vi "Dashboard Main.vi"() -> ()   [LabVIEW 2023]
uses:
  <vilib>/event_ctls.llb/eventvkey.ctl
  <vilib>/Rock Robotics/WPI/Dashboard/WPI_DashboardLogging Global.vi
  <vilib>/Rock Robotics/Network Tables/NT Read Numeric Array.vi
  <vilib>/Rock Robotics/Network Tables/NT Read Boolean.vi
panel:
  in  "Camera Settings Right":T1={"Frame Rate"=30, "Compression"=30, "Size"=1, "DB Camera Config"=FALSE} {"Frame Rate" scale=1.0..30.0; "Compression" scale=100.0..-1.0; "Size" items=["640x480", "320x240", "160x120"]}
  in  "Camera Name Right":string(combo)="No Camera Selection"
  out "Camera Perf":string
  in  "Camera Settings":T1={"Frame Rate"=30, "Compression"=30, "Size"=1, "DB Camera Config"=FALSE} {"Frame Rate" scale=1.0..30.0; "Compression" scale=100.0..-1.0; "Size" items=["640x480", "320x240", "160x120"]}
  in  "TCP":refnum<k5>
  in  "Rec Mode":enum32{"Stop", "Record", "Playback"}(radio)
  out "Robot IP":string
  out "Image Message":string="Timeout in Camera Communications"
  in  "Dashboard Tab":T2(tab)=enum."Custom"
  in  "Select Auto":string(combo)="Select Autonomous ..."
  out "NT Connection":bool
  out "MotorChart R":cluster{"Numeric":dbl, "Numeric":dbl}(graph)
  out "MotorChart L":cluster{"Numeric":dbl, "Numeric":dbl}(graph)
  out "MotorSliders R":cluster{"MotorSlide1":dbl, "MotorSlide2":dbl} {"MotorSlide2" scale=-1.0..1.0 scale format="%#_2e"; "MotorSlide1" scale=-1.0..1.0 scale format="%#_2e"}
  out "MotorSliders L":cluster{"MotorSlide1":dbl, "MotorSlide2":dbl} {"MotorSlide2" scale=-1.0..1.0 scale format="%#_2e"; "MotorSlide1" scale=-1.0..1.0 scale format="%#_2e"}
  out "Gyro":dbl(knob) scale=0.0..360.0
  out "JS1 Z":dbl(slide) scale=-1.0..1.0 scale format="%#_2e"
  out "JS1 Graph":cluster{"X":dbl, "Y":dbl}[](graph)
  out "JS1 Buttons":T3
  out "JS2 Z":dbl(slide) scale=-1.0..1.0 scale format="%#_2e"
  out "JS2 Graph":cluster{"X":dbl, "Y":dbl}[](graph)
  out "JS2 Buttons":T3
  out "Mode":T4(ring)=enum."Auto Disabled"
  out "Right Camera Perf":cluster{"Bandwidth (Mbps)":dbl, "FPS":dbl}
  out "Camera Image Right":T5(plugin-control)
  in  "DB/String 9":string
  in  "DB/String 8":string
  in  "DB/String 7":string
  in  "DB/String 6":string
  in  "DB/String 5":string
  in  "DB/String 4":string
  in  "DB/String 3":string
  in  "DB/String 2":string
  in  "DB/String 1":string
  in  "DB/String 0":string
  in  "DB/Slider 0":dbl(slide) scale=0.0..5.0
  in  "DB/Slider 1":dbl(slide) scale=0.0..5.0
  in  "DB/Slider 2":dbl(slide) scale=0.0..5.0
  in  "DB/Slider 3":dbl(slide) scale=0.0..5.0
  out "DB/LED 3":bool
  out "DB/LED 2":bool
  out "DB/LED 1":bool
  out "DB/LED 0":bool
  in  "DB/Button 3":bool
  in  "DB/Button 2":bool
  in  "DB/Button 1":bool
  in  "DB/Button 0":bool caption="New Name"
  out "Cluster":T6
  in  "Test Slider":dbl(slide) scale=0.0..100.0 scale format="%#_3g"
  in  "On/Off":bool caption="Solenoid"
  in  "Test Name":u16(ring) items=["Select the test to run..."]
  in  "Test Tree":string(tree)
  in  "Motor":cluster{"Value":dbl, "Enable":bool} {"Value" scale=-1.0..1.0 scale format="%#_3g"}
  out "Progress":T7 {"Test Progress" scale=0.0..100.0}
  in  "Rev/Fwd":cluster{"Forward":bool, "Reverse":bool}
  in  "Test Ring":u16(ring) items=["Monochrome", "Color"]
  in  "CheckList":i32(listbox)
  out "Tree":string(tree)
  out "Camera Image":T5(plugin-control)
  out "Background":bool
  in  "Camera Name":string(combo)="No Camera Selection"
  # "HW"
  # "HW"
  # "Joysticks"
  # "Drive Motors"
  # "Front"
  # "Right"
  # "Left"
  # "Back"
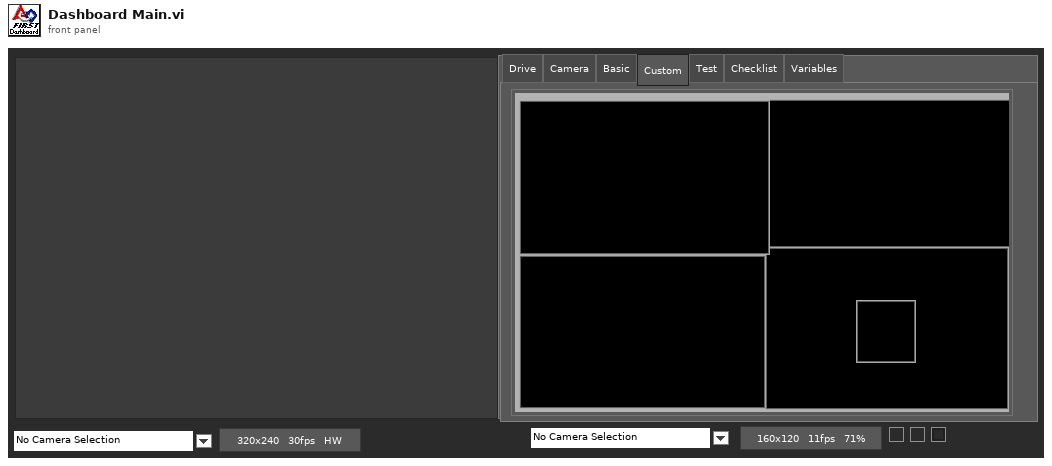
[diagram p1: front panel]
types:
  T1 = cluster{"Frame Rate":i32, "Compression":i32, "Size":u16, "DB Camera Config":bool}
  T2 = enum32{"Drive", "Camera", "Basic", "Custom", "Test", "Checklist", "Variables"}
  T3 = cluster{bool, bool, bool, bool, bool, bool, bool, bool, bool, bool, bool, bool}
  T4 = enum8{"Tele-Op Disabled", "Tele-Op Enabled", "Auto Disabled", "Auto Enabled", "Test Disabled", "Test Enabled", "Disconnected", "No Code", "E-Stop"}
  T5 = typedef "IMAQ Image.ctl" = refnum<image>
  T6 = cluster{"Rotation Align":u32, "Rotation Align 2":u32, "Note Ready":u32, "Y pressed":u32, "Teeth Note":u32}
  T7 = cluster{"Test Progress":u8, "Test Progress Text":string}
  T8 = cluster{"Save Path":path, "Interval (s)":dbl, "Keep":i32}
  T9 = enum32{"Drive", "Camera", "Basic", "Custom", "Test", "Commands", "Checklist", "Variables"}
  T10 = typedef "Image Type" = u32
  T11 = cluster{"Error Strings":string, "Disable Counts":cluster{u16, u16}, "Rail Faults":cluster{u16, u16, u16}, "Robot IP":string, "DB Mode":u8, "Event Info":cluster{"Name":string, "Type":u8, "Number":u16, "Replay":u8}}
  T12 = cluster{"Storage":cluster{"Disk Free":u64, "RAM Block":u32, "RAM free":u32}, "CPU Utilization":cluster{"CPU % ISR":sgl, "CPU % Time Crit":sgl, "CPU % Timed Str":sgl, "CPU % High":sgl, "CPU % Above":sgl, "CPU % Normal":sgl, "CPU % Low":sgl}, "CAN":cluster{"% Bus Utilization":sgl, "Bus Off Cnt":u32, "TX_FIFO Full Cnt":u32, "Receive Error Cnt":u8, "Transmit Error Cnt":u8}, "HID":cluster{"HID Outputs":u32, "Rumble Low":u16, "Rumble High":u16}[]}
  T13 = cluster{"Status bits":cluster{"Test Mode":bool, "Autonomous":bool, "Enabled":bool, "Code Start":bool, "Brownout":bool, "Reserved 2":bool, "Reserved 3":bool, "E-Stop":bool}, "Code Trace":cluster{"Disabled":bool, "TeleOp":bool, "Auto":bool, "Test":bool}, "Controller Type":enum16{"unknown", "cRIO", "roboRio"}, "Code?":enum16{"unknown", "noCode", "code"}, "Battery V":dbl}
  T14 = cluster{"Control Bits":cluster{"TestMode":bool, "Autonomous":bool, "Enabled":bool, "FMS Present":bool, bool, bool, bool, "E-Stop":bool}, "Team Station ":u8, "Countdown":sgl, "Joystick Values":cluster{"Axes":dbl[], "Buttons":bool[], "POVs":i16[]}[]}
  T15 = cluster{"Axes":dbl[], "Buttons":bool[], "POVs":i16[]}[]
  T16 = cluster{"Aligned":u32, "Aligned":u32, "Aligned":u32, "Aligned":u32, "Aligned":u32}
  T17 = cluster{"Axes":dbl[], "Buttons":bool[], "POVs":i16[]}
  T18 = cluster{"Buttons[0]":bool, "Buttons[1]":bool, "Buttons[2]":bool, "Buttons[3]":bool, "Buttons[4]":bool, "Buttons[5]":bool, "Buttons[6]":bool, "Buttons[7]":bool, "Buttons[8]":bool, "Buttons[9]":bool, "Buttons[10]":bool, "Buttons[11]":bool}
  T19 = cluster{"Camera Image":refnum<vi>, "Dashboard Tab":refnum<vi>, "Background":refnum<vi>, "Rec Mode":refnum<vi>, "Test Slider":refnum<vi>, "On/Off ":refnum<vi>, "Test Ring":refnum<vi>, "Rev/Fwd":refnum<vi>, "Test Name":refnum<vi>, "Motor":refnum<vi>, "Progress":refnum<vi>, "CheckList":refnum<vi>, "Tree":refnum<vi>, "Test Tree":refnum<vi>, "Camera Settings":refnum<vi>, "Camera Name":refnum<vi>, "Camera Perf":refnum<vi>, "Camera Settings Right":refnum<vi>, "Camera Name Right":refnum<vi>, "Camera Image Right":refnum<vi>, "Cluster":refnum<vi>}
  T20 = cluster{"Global Rectangle":i32[], "Contours":cluster{"Contour Type":u32, "ROI Type":u32, "Points":i32[]}[]}
  T21 = cluster{"Camera Name":string, string, "Saved DB Images Info":cluster{"Save Path":path, "Interval (s)":dbl, "Keep":i32}}
  T22 = cluster{"Camera Name Right":string, string, "Saved DB Images Info":cluster{"Save Path":path, "Interval (s)":dbl, "Keep":i32}}
  T23 = cluster{"Operation":enum16{"Update", "Clear"}, "Color Box":u32}[]
  T24 = typedef "eventvkey.ctl" = enum16{"ASCII", "Enter", "Return", "Shift", "Ctrl", "Alt", "Cmd", "Opt", "Caps", "NumLock", "Clear", "Break", "Up", "Down", "Left", "Right", "Insert", "Delete", "Home", "End", "PageUp", "PageDown", "Escape", "Help", "Pause", "ScrollLock", "F1", "F2", "F3", "F4", "F5", "F6", "F7", "F8", "F9", "F10", "F11", "F12", "F13", "F14", "F15", "F16", "F17", "F18", "F19", "F20", "F21", "F22", "F23", "F24", "Play", "VolumeUp", "VolumeDown", "Mute", "Two Byte Char"}
  T25 = cluster{"Image Size":bool, "Image Type":bool, "Pixel Value":bool, "ROI Information":bool, "Zoom Factor":bool}
  T26 = cluster{"Operation":enum16{"Update", "Clear"}, "Color Box":u32}
  T27 = cluster{"Shift":bool, "Ctrl":bool, "Alt":bool, "Cmd":bool, "Opt":bool}
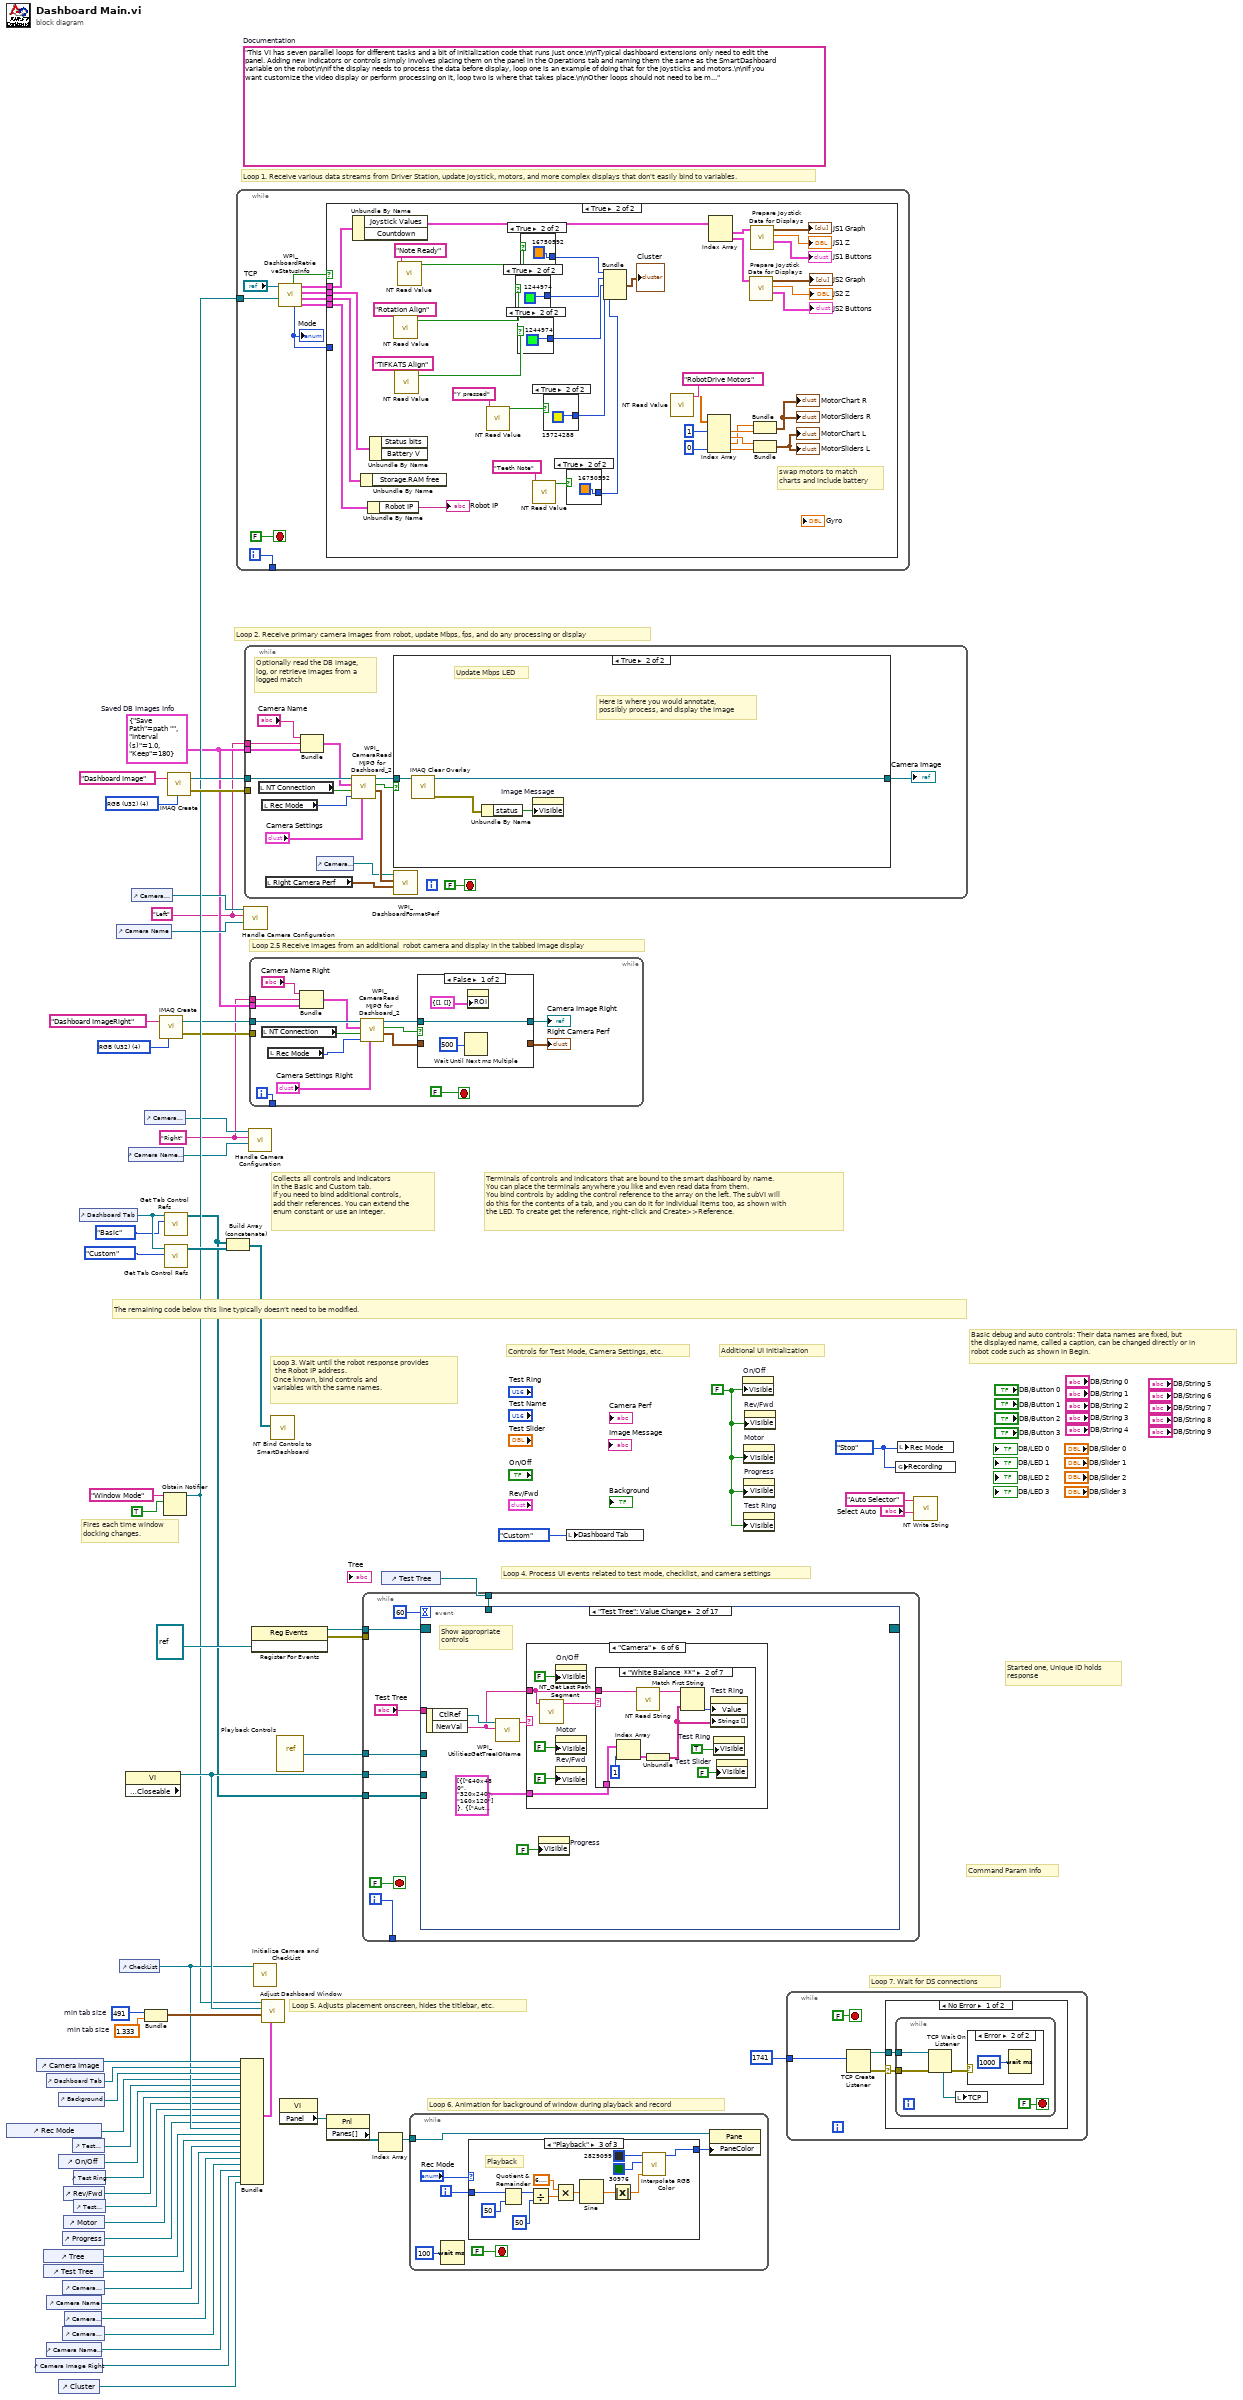
[diagram p0: block diagram]
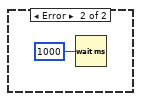
[diagram p4: hidden frame]
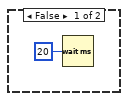
[diagram p5: hidden frame]
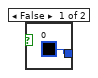
[diagram p6: hidden frame]
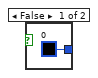
[diagram p7: hidden frame]
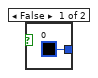
[diagram p8: hidden frame]
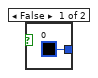
[diagram p9: hidden frame]
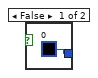
[diagram p10: hidden frame]
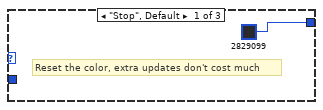
[diagram p11: hidden frame]
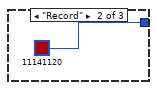
[diagram p12: hidden frame]
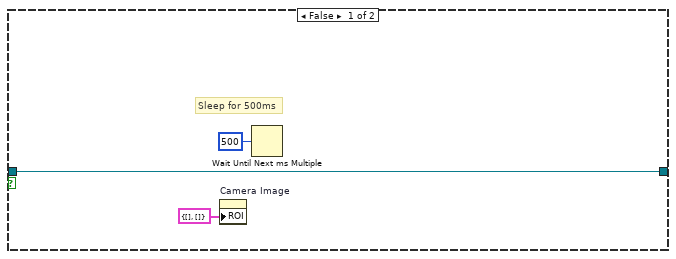
[diagram p13: hidden frame]
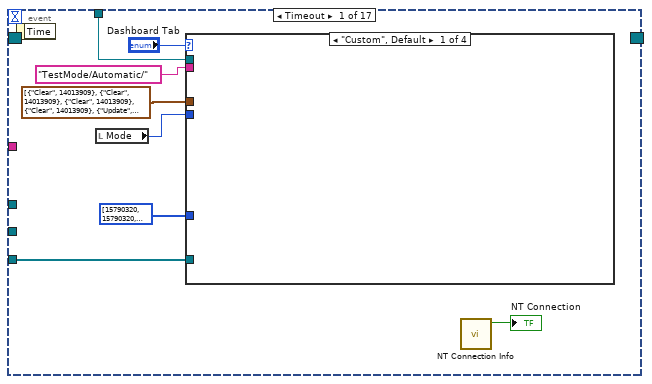
[diagram p14: hidden frame]
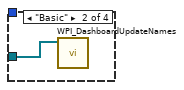
[diagram p15: hidden frame]
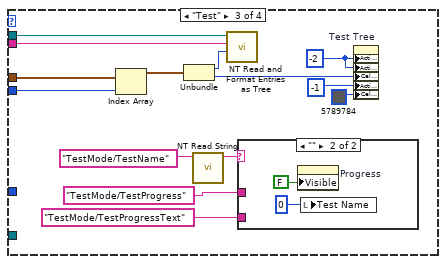
[diagram p16: hidden frame]
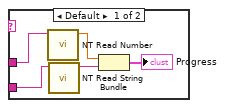
[diagram p17: hidden frame]
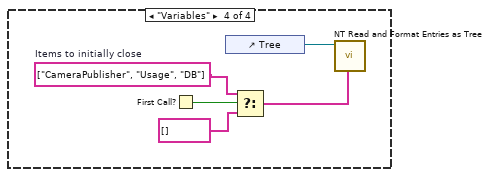
[diagram p18: hidden frame]
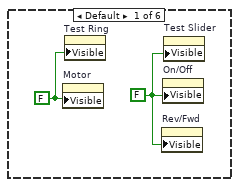
[diagram p19: hidden frame]
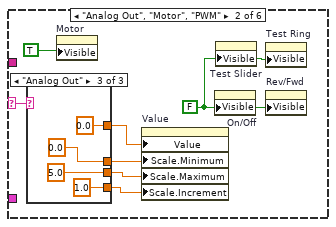
[diagram p20: hidden frame]
diagram:
  w4 = T8 {"Save Path"=path "", "Interval (s)"=1.0, "Keep"=180}  # Saved DB Images Info
  w3 = "Right"
  w2 = "Left"
  w14 = T10 4 items=["Grayscale (U8)", "Grayscale (I16)", "Grayscale (SGL)", "Complex (CSG)", "RGB (U32)", "HSL (U32)", "RGB (U64)"] ("Image Type")
  w43 = 491  # min tab size
  w42 = 1.333  # min tab size
  w50 = enum32{"Stop", "Record", "Playback"}."Stop" ("Rec Mode")
  w27 = FALSE ("Visible")
  (unwired) "This VI has seven parallel loops for different tasks and a bit of initialization code that runs just once.\n\nTypical dashboard extensions only need to edit the panel. Adding new indicators or controls simply involves placing them on the panel in the Operations tab and naming them the same as the SmartDashboard variable on the robot\n\nIf the display needs to process the data before display, loop one is an example of doing that for the joysticks and motors.\n\nIf you want customize the video display or perform processing on it, loop two is where that takes place.\n\nOther loops should not need to be modified. They are pretty standard, and document the task they perform."  # Documentation
  w64 = T10 4 items=["Grayscale (U8)", "Grayscale (I16)", "Grayscale (SGL)", "Complex (CSG)", "RGB (U32)", "HSL (U32)", "RGB (U64)"] ("Image Type")
  # "Loop 2.5 Receive images from an additional  robot camera and display in the tabbed image display"
  # "Command Param Info"
  # "Started one, Unique ID holds\nresponse"
  # "Loop 7. Wait for DS connections"
  # "Basic debug and auto controls: Their data names are fixed, but\nthe displayed name, called a caption, can be changed directly or in\nrobot code such as shown in Begin."
  # "Controls for Test Mode, Camera Settings, etc."
  # "Additional UI Initialization"
  # "Loop 6. Animation for background of window during playback and record"
  # "Fires each time window\ndocking changes."
  # "Collects all controls and indicators\nin the Basic and Custom tab.\nIf you need to bind additional controls,\nadd their references. You can extend the\nenum constant or use an integer."
  # "The remaining code below this line typically doesn't need to be modified."
  # "Loop 4. Process UI events related to test mode, checklist, and camera settings"
  # "Terminals of controls and indicators that are bound to the smart dashboard by name.\nYou can place the terminals anywhere you like and even read data from them.\nYou bind controls by adding the control reference to the array on the left. The subVI will\ndo this for the contents of a tab, and you can do it for individual items too, as shown with\nthe LED. To create get the reference, right-click and Create>>Reference."
  # "Loop 3. Wait until the robot response provides\n the Robot IP address.\nOnce known, bind controls and\nvariables with the same names."
  # "Loop 5. Adjusts placement onscreen, hides the titlebar, etc."
  # "Loop 1. Receive various data streams from Driver Station, update joystick, motors, and more complex displays that don't easily bind to variables."
  # "Loop 2. Receive primary camera images from robot, update Mbps, fps, and do any processing or display"
  n1 = control-ref of="Rec Mode"() -> (w33:refnum<vi>)
  n2 = control-ref of="Camera Image Right"() -> (w7:refnum<vi>)
  n3 = control-ref of="Camera Image"() -> (w45:refnum<vi>)
  n4 = control-ref of="Tree"() -> (w37:refnum<vi>)
  n5 = control-ref of="Test Tree"() -> (w36:refnum<vi>)
  n6 = control-ref of="Dashboard Tab"() -> (w44:refnum<vi>)
  n7 = control-ref of="Camera Name"() -> (w20:refnum<vi>)
  n8 = control-ref of="Camera Name Right"() -> (w8:refnum<vi>)
  n9 = control-ref of="Cluster"() -> (w1:refnum<vi>)
  n10 = control-ref of="Background"() -> (w40:refnum<vi>)
  n11 = control-ref of="On/Off"() -> (w31:refnum<vi>)
  n12 = control-ref of="Progress"() -> (w28:refnum<vi>)
  n13 = control-ref of="Camera Settings"() -> (w21:refnum<vi>)
  n14 = control-ref of="Camera Settings Right"() -> (w9:refnum<vi>)
  n15 = control-ref of="Rev/Fwd"() -> (w29:refnum<vi>)
  n16 = control-ref of="Motor"() -> (w34:refnum<vi>)
  n17 = control-ref of="Camera Perf"() -> (w19:refnum<vi>)
  n18 = control-ref of="Test Slider"() -> (w32:refnum<vi>)
  n19 = control-ref of="Test Ring"() -> (w30:refnum<vi>)
  n20 = control-ref of="Test Name"() -> (w35:refnum<vi>)
  n21 = control-ref of="Dashboard Tab"() -> (w48:refnum<vi>)
  n22 = control-ref of="Camera Name"() -> (w22:refnum<vi>)
  n23 = control-ref of="CheckList"() -> (w38:refnum<vi>)
  n24 = property class="VI" props=["Front Panel.Closeable"]() -> (reference out=w49:refnum<vi>)  [unwired: 2 in, 2 out]
  n25 = control-ref of="Camera Name Right"() -> (w10:refnum<vi>)
  n26 = control-ref of="Camera Settings"() -> (w23:refnum<vi>)
  n27 = control-ref of="Camera Settings Right"() -> (w11:refnum<vi>)
  n28 = Bundle("min tab size"=w43, "min tab size"=w42) -> (w41:cluster{"min tab size":i32, "min tab size":dbl})  [unwired: 1 in]
  n29 = call "IMAQ Create"("Image Name"="Dashboard ImageRight", "Image Type"=w14) -> ("New Image"=w13:T5, "error out"=w12:errorcluster)  [unwired: 2 in, 1 out]
  n30 = Obtain Notifier(name (unnamed)="Window Mode", notification data type=TRUE) -> (notifier out=w26:refnum<notifier>)  [unwired: 2 in, 2 out]
  n31 = call <vilib>:"Get Tab Control Refs.vi"("Page Index"=T9."Basic" ("Dashboard Tab"), "TabControl in"=w48) -> ("ControlsOnPage"=w18:refnum<vi>[])  [unwired: 9 in]
  n32 = call <vilib>:"Get Tab Control Refs.vi"("Page Index"=T9."Custom" ("Dashboard Tab"), "TabControl in"=w48) -> ("ControlsOnPage"=w47:refnum<vi>[])  [unwired: 9 in]
  n33 = call "IMAQ Create"("Image Name"="Dashboard Image", "Image Type"=w64) -> ("New Image"=w62:T5, "error out"=w61:errorcluster)  [unwired: 2 in, 1 out]
  n34 = Build Array (concatenate)(w18, w47) -> (w46:refnum<vi>[])
  n35 = while {
    tunnel: [w73] -> _
    tunnel: w26 -> [w65]
    i -> [w73]
    stop <- FALSE stop-if-true
    n36 = call <vilib>:"WPI_DashboardRetrieveStatusInfo.vi"("Window Mode Notifier"=w65, "TCP Cnx"="TCP") -> ("Power and Errors"=w68:T11, "Robot Metrics"=w71:T12, "Status Info"=w72:T13, "Control Info"=w69:T14, "Robot Mode"=w67:T4, "Process?"=w70:bool)  [unwired: 4 in]
    "Mode" <- w67
    n37 = case shown="True" w70 {
      tunnel: w72 -> [_ w115]
      tunnel: w71 -> [_ w114]
      tunnel: w69 -> [_ w113]
      tunnel: w68 -> [_ w112]
      tunnel: w67 -> [_ _]
      frame False {
        n38 = Wait (ms)(milliseconds to wait=u32 20) -> ()  [unwired: 1 out]
      }
      frame True {
        # "swap motors to match\ncharts and include battery"
        n39 = Unbundle By Name(w113) -> ("Joystick Values"=w103:T15)  [unwired: 1 out]
        n40 = Unbundle By Name(w114) -> ()  [unwired: 1 out]
        n41 = Unbundle By Name(w112) -> ("Robot IP"=→"Robot IP":string)
        n42 = Unbundle By Name(w115) -> ()  [unwired: 2 out]
        n43 = call-poly <vilib>:"NT Read Value.vi"("name"="Rotation Align") -> ("value"=w89:bool)  [unwired: 8 in, 2 out]
        n44 = call-poly <vilib>:"NT Read Value.vi"("name"="TIFKATS Align") -> ("value"=w83:bool)  [unwired: 8 in, 2 out]
        n45 = call-poly <vilib>:"NT Read Value.vi"("name"="Note Ready") -> ("value"=w88:bool)  [unwired: 8 in, 2 out]
        n46 = call-poly <vilib>:"NT Read Value.vi"("name"="Y pressed") -> ("value"=w80:bool)  [unwired: 8 in, 2 out]
        n47 = case shown="True" w89 {
          tunnel: [u32 0 ("Aligned") u32 1244974 ("Aligned")] -> w85
          frame False {
          }
          frame True {
          }
        }
        n48 = case shown="True" w83 {
          tunnel: [u32 0 ("Aligned") u32 1244974 ("Aligned")] -> w82
          frame False {
          }
          frame True {
          }
        }
        n49 = case shown="True" w88 {
          tunnel: [u32 0 ("Aligned") u32 16750592 ("Aligned")] -> w86
          frame False {
          }
          frame True {
          }
        }
        n50 = call-poly <vilib>:"NT Read Value.vi"("name"="Teeth Note") -> ("value"=w77:bool)  [unwired: 8 in, 2 out]
        n51 = case shown="True" w80 {
          tunnel: [u32 0 ("Aligned") u32 15724288 ("Aligned")] -> w79
          frame False {
          }
          frame True {
          }
        }
        n52 = case shown="True" w77 {
          tunnel: [u32 0 ("Aligned") u32 16750592 ("Aligned")] -> w76
          frame False {
          }
          frame True {
          }
        }
        n53 = Bundle("Aligned"=w86, "Aligned"=w85, "Aligned"=w82, "Aligned"=w79, "Aligned"=w76) -> (→"Cluster":T16)  [unwired: 1 in]
        n54 = call-poly <vilib>:"NT Read Value.vi"("name"="RobotDrive Motors" ("Name")) -> ("value"=w93:dbl[])  [unwired: 8 in, 2 out]
        n55 = Index Array(array=w93, index #1=1, index #4=0) -> (element #1=w107:dbl, element #2=w108:dbl, element #3=w106:dbl, element #4=w111:dbl)  [unwired: 2 in]
        n56 = Index Array(array=w103) -> (element #1=w102:T17, element #2=w98:T17)  [unwired: 2 in]
        n57 = call "Prepare Joystick Data for Displays.vi"("Joystick Values"=w98) -> ("Buttons"=→"JS2 Buttons":T18, "Z Axis"=→"JS2 Z":dbl, "Cartesian Data"=→"JS2 Graph":cluster{"X axis":dbl, "X axis":dbl}[])  [unwired: 8 in]
        n58 = call "Prepare Joystick Data for Displays.vi"("Joystick Values"=w102) -> ("Buttons"=→"JS1 Buttons":T18, "Z Axis"=→"JS1 Z":dbl, "Cartesian Data"=→"JS1 Graph":cluster{"X axis":dbl, "X axis":dbl}[])  [unwired: 8 in]
        n59 = Bundle("Numeric"=w106, "Numeric"=w107) -> (→"MotorChart R" →"MotorSliders R":cluster{"Numeric":dbl, "Numeric":dbl})  [unwired: 1 in]
        n60 = Bundle("Numeric"=w108, "Numeric"=w111) -> (→"MotorChart L" →"MotorSliders L":cluster{"Numeric":dbl, "Numeric":dbl})  [unwired: 1 in]
      }
    }
  }
  n61 = Bundle("Camera Image"=w45, "Dashboard Tab"=w44, "Background"=w40, "Rec Mode"=w33, "Test Slider"=w32, "On/Off"=w31, "Test Ring"=w30, "Rev/Fwd"=w29, "Test Name"=w35, "Motor"=w34, "Progress"=w28, "CheckList"=w38, "Tree"=w37, "Test Tree"=w36, "Camera Settings"=w21, "Camera Name"=w20, "Camera Perf"=w19, "Camera Settings Right"=w9, "Camera Name Right"=w8, "Camera Image Right"=w7, "Cluster"=w1) -> (w39:T19)  [unwired: 1 in]
  n62 = call "Handle Camera Configuration.vi"("CameraNameRef"=w22, "Display Name"=w2, "ClusterRef"=w23) -> ()  [unwired: 9 in]
  n63 = while {
    tunnel: w62 -> [w139]
    tunnel: w61 -> [_]
    tunnel: w4 -> [w132]
    tunnel: w2 -> [w129]
    stop <- FALSE stop-if-true
    # "Optionally read the DB image,\nlog, or retrieve images from a\nlogged match"
    n64 = local read "NT Connection"() -> (w133:bool)
    n65 = local read "Rec Mode"() -> (w136:enum32{"Stop", "Record", "Playback"})
    n66 = local read "Right Camera Perf"() -> (w127:cluster{"Bandwidth (Mbps)":dbl, "FPS":dbl})
    n67 = Bundle("Camera Name"="Camera Name", w129, "Saved DB Images Info"=w132) -> (w131:T21)  [unwired: 1 in]
    n68 = control-ref of="Camera Perf"() -> (w126:refnum<vi>)
    n69 = call <vilib>:"WPI_CameraRead MJPG for Dashboard_2.vi"("Camera Settings"="Camera Settings", "Rec Mode"=w136, "NT Connection"=w133, "Capture Info"=w131, "Image in"=w139) -> ("perf info"=w128:cluster{"Bandwidth (Mbps)":dbl, "fps":dbl}, "Active"=w137:bool, "Image\\ out"=w138:T5)  [unwired: 4 in]
    n70 = case shown="True" w137 {
      tunnel: w138 -> [w142 w145]
      tunnel: [w142 w144] -> w134
      frame False {
        # "Sleep for 500ms"
        n71 = property on="Camera Image" class="ImageControl"("ROI"=T20 {"Global Rectangle"=[], "Contours"=[]}) -> ()  [unwired: 2 in, 2 out]
        n72 = Wait Until Next ms Multiple(millisecond multiple=u32 500) -> ()  [unwired: 1 out]
      }
      frame True {
        # "Here is where you would annotate,\npossibly process, and display the image"
        # "Update Mbps LED"
        n73 = call "IMAQ Clear Overlay"("Image"=w145) -> ("error out"=w146:errorcluster, "Image Out"=w144:T5)  [unwired: 2 in, 7 out]
        n74 = Unbundle By Name(w146) -> ("status"=w147:bool)
        n75 = property on="Image Message" class="Str"("Visible"=w147) -> ()  [unwired: 2 in, 2 out]
      }
    }
    "Camera Image" <- w134
    n76 = call <vilib>:"WPI_DashboardFormatPerf.vi"("Right Camera Perf"=w127, "Performance"=w128, "String in"=w126) -> ()  [unwired: 9 in]
  }
  n77 = call "Handle Camera Configuration.vi"("CameraNameRef"=w10, "Display Name"=w3, "ClusterRef"=w11) -> ()  [unwired: 9 in]
  n78 = while {
    tunnel: w13 -> [w162]
    tunnel: w12 -> [_]
    tunnel: [w157] -> _
    tunnel: w4 -> [w153]
    tunnel: w3 -> [w150]
    i -> [w157]
    stop <- FALSE stop-if-true
    n79 = local read "NT Connection"() -> (w154:bool)
    n80 = local read "Rec Mode"() -> (w161:enum32{"Stop", "Record", "Playback"})
    n81 = Bundle("Camera Name Right"="Camera Name Right", w150, "Saved DB Images Info"=w153) -> (w152:T22)  [unwired: 1 in]
    n82 = call <vilib>:"WPI_CameraRead MJPG for Dashboard_2.vi"("Camera Settings"="Camera Settings Right", "Rec Mode"=w161, "NT Connection"=w154, "Capture Info"=w152, "Image in"=w162) -> ("perf info"=w148:cluster{"Bandwidth (Mbps)":dbl, "fps":dbl}, "Active"=w156:bool, "Image\\ out"=w159:T5)  [unwired: 4 in]
    n83 = case shown="False" w156 {
      tunnel: w159 -> [w164 w167]
      tunnel: [w164 w167] -> w155
      tunnel: [_ w166] -> w149
      tunnel: w148 -> [_ w166]
      frame False {
        n84 = Wait Until Next ms Multiple(millisecond multiple=u32 500) -> ()  [unwired: 1 out]
        n85 = property on="Camera Image Right" class="ImageControl"("ROI"=T20 {"Global Rectangle"=[], "Contours"=[]}) -> ()  [unwired: 2 in, 2 out]
      }
      frame True {
      }
    }
    "Camera Image Right" <- w155
    "Right Camera Perf" <- w149
  }
  n86 = register-events(refnum<vi> refnum) -> (reference out=w53:refnum<event-registration>, error out=w52:errorcluster)  [unwired: 2 in]
  n87 = call "Initialize Camera and CheckList.vi"("ListBox in"=w38) -> ()  [unwired: 11 in]
  n88 = call "Adjust Dashboard Window.vi"("Sizing Refnums"=w39, "Size Constraints"=w41, "VI"=w49, "WIn Mode"=w26) -> ()  [unwired: 8 in]
  n89 = call <vilib>:"NT Bind Controls to SmartDashboard.vi"("Bound Control Refs"=w46) -> ()  [unwired: 11 in]
  n90 = vi-ref "Playback Controls.vi"() -> (w54:refnum<vi>)
  n91 = property class="VI"() -> ("Panel"=w56:refnum<vi>)  [unwired: 2 in, 2 out]
  n92 = property class="Pnl"(reference=w56) -> ("Panes[]"=w57:refnum<vi>[])  [unwired: 1 in, 2 out]
  n93 = Index Array(array=w57) -> (element=w55:refnum<vi>)  [unwired: 1 in]
  n94 = control-ref of="Test Tree"() -> (w58:refnum<vi>)
  n95 = while {
    tunnel: [w173] -> _
    tunnel: w58 -> [w172]
    tunnel: w54 -> [w171]
    tunnel: w53 -> [w170]
    tunnel: w52 -> [_]
    tunnel: w49 -> [w169]
    tunnel: w18 -> [w168]
    i -> [w173]
    stop <- FALSE stop-if-true
    n96 = event shown="[1] \"Test Tree\": Value Change" {
      selector: w170 -> [_ _ _ _ _ _ _ _ _ _ _ _ _ _ _ _ _]
      dyn-events: [_ _ _ _ _ _ _ _ _ _ _ _ _ w378 _ _ _] -> _
      timeout: u32 60 ("milliseconds to wait") -> [_ _ _ _ _ _ _ _ _ _ _ _ _ _ _ _ _]
      tunnel: w172 -> [w183 _ _ _ _ _ _ _ _ _ _ _ _ _ _ _ _]
      tunnel: "Test Tree" -> [_ _ _ _ _ _ _ _ w351 w358 w359 w362 w369 _ _ _ _]
      tunnel: w171 -> [_ _ _ _ _ _ _ _ _ _ _ _ _ w380 _ w395 _]
      tunnel: w169 -> [_ _ _ _ _ _ _ _ _ _ _ _ _ w376 _ _ _]
      tunnel: w168 -> [w178 _ _ _ _ _ _ _ _ _ _ _ _ _ _ _ _]
      event Timeout {
        n97 = event-data() -> ()  [unwired: 1 in, 1 out]
        n98 = local read "Mode"() -> (w181:T4)
        n99 = case shown="\"Custom\", Default" "Dashboard Tab" {
          tunnel: w183 -> [_ _ w199 _]
          tunnel: "TestMode/Automatic/" ("Name Pattern") -> [_ _ w198 _]
          tunnel: T23 [{"Operation"=enum."Clear", "Color Box"=14013909}, {"Operation"=enum."Clear", "Color Box"=14013909}, {"Operation"=enum."Clear", "Color Box"=14013909}, {"Operation"=enum."Clear", "Color Box"=14013909}, {"Operation"=enum."Update", "Color Box"=14013909}, {"Operation"=enum."Update", "Color Box"=16777215}, {"Operation"=enum."Clear", "Color Box"=14013909}, {"Operation"=enum."Clear", "Color Box"=14013909}, {"Operation"=enum."Clear", "Color Box"=14013909}] -> [_ _ w191 _]
          tunnel: w181 -> [_ _ w190 _]
          tunnel: u32[] [15790320, 15790320, 15790320, 15790320, 16777215, 16777215, 15790320, 15790320, 15790320] -> [_ _ _ _]
          tunnel: w178 -> [_ w185 _ _]
          frame "Custom", Default {
          }
          frame "Basic" {
            n100 = call <vilib>:"WPI_DashboardUpdateNames.vi"("Controls on Tab"=w185) -> ()  [unwired: 11 in]
          }
          frame "Test" {
            w197 = -2 ("Active Item:Row Number")
            n101 = Index Array(array=w191, index=w190) -> (element=w192:T26)
            n102 = Unbundle(w192) -> ("Operation"=w193:enum16{"Update", "Clear"}, "Color Box"=w194:u32)
            n103 = call <vilib>:"NT Read String.vi"("name"="TestMode/TestName" ("Name")) -> ("value"=w188:string)  [unwired: 8 in, 2 out]
            n104 = call <vilib>:"NT Read and Format Entries as Tree.vi"("Operation"=w193, "Name Pattern"=w198, "Tree Refnum"=w199) -> ()  [unwired: 7 in, 2 out]
            n105 = case shown="\"\"" w188 {
              tunnel: "TestMode/TestProgress" ("Name") -> [w201 _]
              tunnel: "TestMode/TestProgressText" ("Name") -> [w200 _]
              frame Default {
                n106 = call <vilib>:"NT Read Number.vi"("name"=w201) -> ("value"=w202:dbl)  [unwired: 8 in, 2 out]
                n107 = call <vilib>:"NT Read String.vi"("name"=w200) -> ("value"=w203:string)  [unwired: 8 in, 2 out]
                n108 = Bundle("value"=w202, "value"=w203) -> (→"Progress":cluster{"value":dbl, "value":string})  [unwired: 1 in]
              }
              frame "" {
                n109 = property on="Progress" class="Clust (strict)"("Visible"=FALSE) -> ()  [unwired: 2 in, 2 out]
                n110 = local write "Test Name"(u16 0) -> ()
              }
            }
            n111 = property on="Test Tree" class="Tree (strict)"("Active Item Row Number"=w197, "ActiveColNum"=w197, "CellBG"=w194, "Active Item Row Number"=-1 ("Active Item:Row Number"), "CellBG"=u32 5789784 ("Color Box")) -> ()  [unwired: 2 in, 2 out]
          }
          frame "Variables" {
            w209 = string[] ["CameraPublisher", "Usage", "DB"]  # Items to initially close
            n112 = First Call?() -> (First Call?: T/F=w210:bool)
            n113 = control-ref of="Tree"() -> (w211:refnum<vi>)
            n114 = Select(t=w209, s=w210, f=string[] []) -> (s? t:f=w207:string[])
            n115 = call <vilib>:"NT Read and Format Entries as Tree.vi"("Tags to  Close"=w207, "Tree Refnum"=w211) -> ()  [unwired: 8 in, 2 out]
          }
        }
        n116 = call <vilib>:"NT Connection Info.vi"() -> ("Connected"=→"NT Connection":bool)  [unwired: 11 in]
      }
      event "Test Tree": Value Change {
        # "Show appropriate\ncontrols"
        n117 = event-data() -> ("CtlRef"=w215:refnum<vi>, "NewVal"=w213:string)  [unwired: 1 in]
        n118 = call <vilib>:"WPI_UtilitiesGetTreeIOName.vi"("NewVal"=w213, "TreeControl in"=w215) -> ("I/O Name"=w216:string)  [unwired: 9 in]
        n119 = case shown="\"Camera\"" w216 {
          selector: w216 -> [_ w223 _ w245 w254 _]
          tunnel: w213 -> [_ _ w242 w244 _ w261]
          tunnel: cluster{string[]}[] [{["640x480", "320x240", "160x120"]}, {["Auto", "Fixed indoor", "Fixed outdoor 1", "Fixed outdoor 2", "Fixed fluorescent 1", "Fixed fluorescent 2", "Hold current"]}, {["Auto", "Flicker-free 50 Hz", "Flicker-free 60 Hz", "Hold current"]}, {["None", "Prioritize frame rate", "Prioritize image quality"]}, {["Monochrome", "Color"]}] -> [_ _ _ _ _ w260]
          frame Default {
            w218 = FALSE ("Visible")
            w217 = FALSE ("Visible")
            n120 = property on="Motor" class="Clust (strict)"("Visible"=w217) -> ()  [unwired: 2 in, 2 out]
            n121 = property on="Test Ring" class="Ring (strict)"("Visible"=w217) -> ()  [unwired: 2 in, 2 out]
            n122 = property on="Rev/Fwd" class="Clust (strict)"("Visible"=w218) -> ()  [unwired: 2 in, 2 out]
            n123 = property on="On/Off" class="Bool (strict)"("Visible"=w218) -> ()  [unwired: 2 in, 2 out]
            n124 = property on="Test Slider" class="Slide (strict)"("Visible"=w218) -> ()  [unwired: 2 in, 2 out]
          }
          frame "Analog Out", "Motor", "PWM" {
            w224 = FALSE ("Visible")
            n125 = case shown="\"Analog Out\"" w223 {
              tunnel: [1.0 ("Value") -1.0 ("Value") 0.0 ("Value")] -> w222
              tunnel: [255.0 ("Value") 1.0 ("Value") 5.0 ("Value")] -> w221
              tunnel: [128.0 ("Value") 0.0 ("Value") 0.0 ("Value")] -> w220
              tunnel: [64.0 ("Value") 0.5 ("Value") 1.0 ("Value")] -> w219
              frame "PWM" {
              }
              frame "Motor", Default {
              }
              frame "Analog Out" {
              }
            }
            n126 = property on="Motor" class="Clust (strict)"("Visible"=TRUE) -> ()  [unwired: 2 in, 2 out]
            n127 = property on="Value" class="Slide (strict)"("Value"=w220, "Scale.Minimum"=w222, "Scale.Maximum"=w221, "Scale.Increment"=w219) -> ()  [unwired: 2 in, 2 out]
            n128 = property on="On/Off" class="Bool (strict)"("Visible"=w224) -> ()  [unwired: 2 in, 2 out]
            n129 = property on="Test Slider" class="Slide (strict)"("Visible"=w224) -> ()  [unwired: 2 in, 2 out]
            n130 = property on="Test Ring" class="Ring (strict)"("Visible"=w224) -> ()  [unwired: 2 in, 2 out]
            n131 = property on="Rev/Fwd" class="Clust (strict)"("Visible"=w224) -> ()  [unwired: 2 in, 2 out]
          }
          frame "Servo" {
            w240 = FALSE ("Visible")
            n132 = call <vilib>:"NT Read Number.vi"("name"=w242) -> ("value"=w241:dbl)  [unwired: 8 in, 2 out]
            n133 = property on="Test Slider" class="Slide (strict)"("Visible"=TRUE, "Scale.Maximum"=170.0 ("Scale.Range:Maximum")) -> ()  [unwired: 2 in, 2 out]
            n134 = local write "Test Slider"(w241) -> ()
            n135 = property on="Motor" class="Clust (strict)"("Visible"=w240) -> ()  [unwired: 2 in, 2 out]
            n136 = property on="Rev/Fwd" class="Clust (strict)"("Visible"=w240) -> ()  [unwired: 2 in, 2 out]
            n137 = property on="On/Off" class="Bool (strict)"("Visible"=w240) -> ()  [unwired: 2 in, 2 out]
            n138 = property on="Test Ring" class="Ring (strict)"("Visible"=w240) -> ()  [unwired: 2 in, 2 out]
          }
          frame "Relay", "Solenoid" {
            w243 = FALSE ("Visible")
            n139 = property on="Motor" class="Clust (strict)"("Visible"=w243) -> ()  [unwired: 2 in, 2 out]
            n140 = property on="Test Slider" class="Slide (strict)"("Visible"=w243) -> ()  [unwired: 2 in, 2 out]
            n141 = Search and Replace String(input string=w244, search string="/Value  **", replace string="/Direction") -> (result string=w250:string)  [unwired: 5 in, 3 out]
            n142 = property on="Test Ring" class="Ring (strict)"("Visible"=w243) -> ()  [unwired: 2 in, 2 out]
            n143 = call <vilib>:"NT Read String.vi"("name"=w250) -> ("value"=w248:string)  [unwired: 8 in, 2 out]
            n144 = Equal?(x="Both directions", y=w248) -> (x = y?=w246:bool)
            n145 = Not(x=w246) -> (.not. x?=w247:bool)
            n146 = property on="Rev/Fwd" class="Clust (strict)"("Visible"=w246) -> ()  [unwired: 2 in, 2 out]
            n147 = property on="On/Off" class="Bool (strict)"("Visible"=w247, "Caption.Text"=w245) -> ()  [unwired: 2 in, 2 out]
          }
          frame "Compressor", "Digital Out" {
            w253 = FALSE ("Visible")
            # "Get direction and finish"
            n148 = property on="Motor" class="Clust (strict)"("Visible"=w253) -> ()  [unwired: 2 in, 2 out]
            n149 = property on="Test Slider" class="Slide (strict)"("Visible"=w253) -> ()  [unwired: 2 in, 2 out]
            n150 = property on="Test Ring" class="Ring (strict)"("Visible"=w253) -> ()  [unwired: 2 in, 2 out]
            n151 = property on="On/Off" class="Bool (strict)"("Visible"=TRUE, "Caption.Text"=w254) -> ()  [unwired: 2 in, 2 out]
            n152 = property on="Rev/Fwd" class="Clust (strict)"("Visible"=FALSE) -> ()  [unwired: 2 in, 2 out]
          }
          frame "Camera" {
            n153 = call <vilib>:"NT_Get Last Path Segment.vi"("String in"=w261) -> ("String out"=w262:string)  [unwired: 10 in]
            n154 = property on="On/Off" class="Bool (strict)"("Visible"=FALSE) -> ()  [unwired: 2 in, 2 out]
            n155 = property on="Motor" class="Clust (strict)"("Visible"=FALSE) -> ()  [unwired: 2 in, 2 out]
            n156 = property on="Rev/Fwd" class="Clust (strict)"("Visible"=FALSE) -> ()  [unwired: 2 in, 2 out]
            n157 = case shown="\"White Balance  **\"" w262 {
              tunnel: w261 -> [w268 w277 w286 w295 w304 _ w310]
              tunnel: w260 -> [w266 w274 w283 w292 w301 _ _]
              frame "Size  **" {
                n158 = Index Array(array=w266) -> (element=w265:cluster{string[]})  [unwired: 1 in]
                n159 = call <vilib>:"NT Read String.vi"("name"=w268) -> ("value"=w267:string)  [unwired: 8 in, 2 out]
                n160 = Unbundle(w265) -> (w263:string[])
                n161 = Match First String(2:w263, 3:w267) -> (0:w264:i32)  [unwired: 1 out]
                n162 = property on="Test Ring" class="Ring (strict)"("Value"=w264, "Strings []"=w263) -> ()  [unwired: 2 in, 2 out]
                n163 = property on="Test Ring" class="Ring (strict)"("Visible"=TRUE) -> ()  [unwired: 2 in, 2 out]
                n164 = property on="Test Slider" class="Slide (strict)"("Visible"=FALSE) -> ()  [unwired: 2 in, 2 out]
              }
              frame "White Balance  **" {
                n165 = Index Array(array=w274, index=1) -> (element=w275:cluster{string[]})
                n166 = call <vilib>:"NT Read String.vi"("name"=w277) -> ("value"=w276:string)  [unwired: 8 in, 2 out]
                n167 = Unbundle(w275) -> (w272:string[])
                n168 = Match First String(2:w272, 3:w276) -> (0:w271:i32)  [unwired: 1 out]
                n169 = property on="Test Ring" class="Ring (strict)"("Value"=w271, "Strings []"=w272) -> ()  [unwired: 2 in, 2 out]
                n170 = property on="Test Ring" class="Ring (strict)"("Visible"=TRUE) -> ()  [unwired: 2 in, 2 out]
                n171 = property on="Test Slider" class="Slide (strict)"("Visible"=FALSE) -> ()  [unwired: 2 in, 2 out]
              }
              frame "Exposure  **" {
                n172 = Index Array(array=w283, index=2) -> (element=w284:cluster{string[]})
                n173 = call <vilib>:"NT Read String.vi"("name"=w286) -> ("value"=w285:string)  [unwired: 8 in, 2 out]
                n174 = Unbundle(w284) -> (w280:string[])
                n175 = Match First String(2:w280, 3:w285) -> (0:w281:i32)  [unwired: 1 out]
                n176 = property on="Test Ring" class="Ring (strict)"("Value"=w281, "Strings []"=w280) -> ()  [unwired: 2 in, 2 out]
                n177 = property on="Test Ring" class="Ring (strict)"("Visible"=TRUE) -> ()  [unwired: 2 in, 2 out]
                n178 = property on="Test Slider" class="Slide (strict)"("Visible"=FALSE) -> ()  [unwired: 2 in, 2 out]
              }
              frame "Exposure Priority  **" {
                n179 = Index Array(array=w292, index=3) -> (element=w293:cluster{string[]})
                n180 = call <vilib>:"NT Read String.vi"("name"=w295) -> ("value"=w294:string)  [unwired: 8 in, 2 out]
                n181 = Unbundle(w293) -> (w289:string[])
                n182 = Match First String(2:w289, 3:w294) -> (0:w290:i32)  [unwired: 1 out]
                n183 = property on="Test Ring" class="Ring (strict)"("Value"=w290, "Strings []"=w289) -> ()  [unwired: 2 in, 2 out]
                n184 = property on="Test Ring" class="Ring (strict)"("Visible"=TRUE) -> ()  [unwired: 2 in, 2 out]
                n185 = property on="Test Slider" class="Slide (strict)"("Visible"=FALSE) -> ()  [unwired: 2 in, 2 out]
              }
              frame "Color Enable  **" {
                n186 = Index Array(array=w301, index=4) -> (element=w302:cluster{string[]})
                n187 = call <vilib>:"NT Read String.vi"("name"=w304) -> ("value"=w303:string)  [unwired: 8 in, 2 out]
                n188 = Unbundle(w302) -> (w298:string[])
                n189 = Match First String(2:w298, 3:w303) -> (0:w299:i32)  [unwired: 1 out]
                n190 = property on="Test Ring" class="Ring (strict)"("Value"=w299, "Strings []"=w298) -> ()  [unwired: 2 in, 2 out]
                n191 = property on="Test Ring" class="Ring (strict)"("Visible"=TRUE) -> ()  [unwired: 2 in, 2 out]
                n192 = property on="Test Slider" class="Slide (strict)"("Visible"=FALSE) -> ()  [unwired: 2 in, 2 out]
              }
              frame Default {
                n193 = property on="Test Ring" class="Ring (strict)"("Visible"=FALSE) -> ()  [unwired: 2 in, 2 out]
                n194 = property on="Test Slider" class="Slide (strict)"("Visible"=FALSE) -> ()  [unwired: 2 in, 2 out]
              }
              frame "Brightness  **", "Color Level  **", "Compression  **", "FPS  **", "Sharpness  **" {
                n195 = call <vilib>:"NT Read Number.vi"("name"=w310) -> ("value"=w309:dbl)  [unwired: 8 in, 2 out]
                n196 = local write "Test Slider"(w309) -> ()
                n197 = property on="Test Ring" class="Ring (strict)"("Visible"=FALSE) -> ()  [unwired: 2 in, 2 out]
                n198 = property on="Test Slider" class="Slide (strict)"("Visible"=TRUE, "Scale.Maximum"=100.0 ("Scale.Range:Maximum")) -> ()  [unwired: 2 in, 2 out]
              }
            }
          }
        }
        n199 = property on="Progress" class="Clust (strict)"("Visible"=FALSE) -> ()  [unwired: 2 in, 2 out]
      }
      event "Test Name": Mouse Enter {
        # "Populate the ring with the list of tests"
        n200 = event-data() -> ()  [unwired: 1 in, 1 out]
        n201 = call <vilib>:"NT Read String Array.vi"("name"="TestMode/TestList" ("Name")) -> ("value"=w317:string[])  [unwired: 8 in, 2 out]
        n202 = Build Array (concatenate)("Select the test to run...", w317) -> (w316:string[])
        n203 = property on="Test Name" class="Ring (strict)"("Strings []"=w316) -> ()  [unwired: 2 in, 2 out]
      }
      event "Test Name": Value Change {
        w318 = FALSE ("Visible")
        # "Tell the robot the test name to run"
        n204 = event-data() -> ("NewVal"=w322:u16)  [unwired: 1 in]
        n205 = property on="Test Name" class="Ring (strict)"() -> ("Strings []"=w323:string[])  [unwired: 2 in, 2 out]
        n206 = local write "Progress"(T7 {"Test Progress"=0, "Test Progress Text"=""} ("Progress")) -> ()
        n207 = Index Array(array=w323, index=w322) -> (element=w321:string)
        n208 = call <vilib>:"NT Write String.vi"("value"=w321, "name"="TestMode/TestName" ("Name")) -> ()  [unwired: 9 in, 1 out]
        n209 = property on="Progress" class="Clust (strict)"("Visible"=TRUE) -> ()  [unwired: 2 in, 2 out]
        n210 = property on="Motor" class="Clust (strict)"("Visible"=w318) -> ()  [unwired: 2 in, 2 out]
        n211 = property on="Test Slider" class="Slide (strict)"("Visible"=w318) -> ()  [unwired: 2 in, 2 out]
        n212 = property on="On/Off" class="Bool (strict)"("Visible"=w318) -> ()  [unwired: 2 in, 2 out]
        n213 = property on="Rev/Fwd" class="Clust (strict)"("Visible"=w318) -> ()  [unwired: 2 in, 2 out]
        n214 = property on="Test Ring" class="Ring (strict)"("Visible"=w318) -> ()  [unwired: 2 in, 2 out]
      }
      event "Select Auto": Mouse Enter {
        # "Populate the combo box with the list of autonomous options"
        n215 = event-data() -> ()  [unwired: 1 in, 1 out]
        n216 = call <vilib>:"NT Read String Array.vi"("name"="Auto List" ("Name")) -> ("value"=w325:string[])  [unwired: 8 in, 2 out]
        n217 = property on="Select Auto" class="CmbBox"("Strings[]"=w325) -> ()  [unwired: 2 in, 2 out]
      }
      event "Select Auto": Value Change {
        # "User modified the Auto Selection. Write to NT variable so robot knows."
        n218 = event-data() -> ("NewVal"=w327:string)  [unwired: 1 in]
        n219 = call <vilib>:"NT Write String.vi"("value"=w327, "name"="Auto Selector" ("Name")) -> ()  [unwired: 9 in, 1 out]
      }
      event "CheckList": Double Click {
        # "Shift clears all"
        # "Update symbols on the listbox"
        n220 = event-data() -> ("PlatMods.Shift"=w329:bool, "Row"=w331:i32)  [unwired: 1 in]
        n221 = case shown="True" w329 {
          tunnel: w331 -> [w335 _]
          tunnel: 1 -> [w334 _]
          frame False {
            n222 = property on="CheckList" class="LstBox (strict)"() -> ("Item Symbols"=w333:i32[])  [unwired: 2 in, 2 out]
            n223 = Replace Array Subset(array=w333, new element=w334, index=w335) -> (w332:i32[])
            n224 = property on="CheckList" class="LstBox (strict)"("Item Symbols"=w332) -> ()  [unwired: 2 in, 2 out]
          }
          frame True {
            w336 = 0 ("Top Row")
            n225 = property on="CheckList" class="LstBox (strict)"() -> ("Number of Rows"=w338:u32)  [unwired: 2 in, 2 out]
            n226 = Initialize Array(0, w338) -> (w337:i32[])
            n227 = property on="CheckList" class="LstBox (strict)"("Top Row"=w336, "Value"=w336, "Item Symbols"=w337) -> ()  [unwired: 2 in, 2 out]
          }
        }
      }
      event "CheckList": Key Down {
        # "Update symbols on the listbox\nLeft and right keys check and uncheck"
        n228 = event-data() -> ("VKey"=w341:T24)  [unwired: 1 in]
        n229 = case shown="\"Left\", \"Right\"" w341 {
          selector: w341 -> [w346 _]
          tunnel: eventvkey."Left" ("VKey") -> [w344 _]
          frame "Left", "Right" {
            n230 = Equal?(x=w344, y=w346) -> (x = y?=w345:bool)
            n231 = Select(t=0, s=w345, f=1) -> (s? t:f=w347:i32)
            n232 = property on="CheckList" class="LstBox (strict)"() -> ("Item Symbols"=w350:i32[])  [unwired: 2 in, 2 out]
            n233 = Replace Array Subset(array=w350, new element=w347, index="CheckList") -> (w349:i32[])
            n234 = property on="CheckList" class="LstBox (strict)"("Item Symbols"=w349) -> ()  [unwired: 2 in, 2 out]
          }
          frame Default {
          }
        }
      }
      event "Motor.Enable": Value Change {
        # "When the test mode otor enable helper is set, update that\ntree row item's value"
        n235 = event-data() -> ("NewVal"=w355:bool)  [unwired: 1 in]
        n236 = Unbundle("Motor") -> ("Value"=w354:dbl)  [unwired: 1 out]
        n237 = Select(t=w354, s=w355, f=0.0) -> (s? t:f=w352:dbl)
        n238 = call <vilib>:"NT Write Number.vi"("value"=w352, "name"=w351) -> ()  [unwired: 9 in, 1 out]
      }
      event "Test Slider": Value Change {
        # "When the test mode slider helper is set, update that\ntree row item's value"
        n239 = event-data() -> ("NewVal"=w357:dbl)  [unwired: 1 in]
        n240 = call <vilib>:"NT Write Number.vi"("value"=w357, "name"=w358) -> ()  [unwired: 9 in, 1 out]
      }
      event "On/Off": Value Change {
        # "When the test mode on/off helper value is set, update that\ntree row item's value"
        n241 = event-data() -> ("NewVal"=w361:bool)  [unwired: 1 in]
        n242 = Boolean To (0,1)(Boolean=w361) -> (0, 1=w360:i16)
        n243 = call <vilib>:"NT Write Number.vi"("value"=w360, "name"=w359) -> ()  [unwired: 9 in, 1 out]
      }
      event "Rev/Fwd": Value Change {
        # "When the test mode helper value for relays is set, update that\ntree row item's value"
        n244 = event-data() -> ("NewVal.Forward"=w368:bool, "NewVal.Reverse"=w367:bool)  [unwired: 1 in]
        n245 = Boolean To (0,1)(Boolean=w368) -> (0, 1=w364:i16)
        n246 = Boolean To (0,1)(Boolean=w367) -> (0, 1=w366:i16)
        n247 = Negate(x=w366) -> (-x=w365:i16)
        n248 = Add(x=w364, y=w365) -> (x+y=w363:i16)
        n249 = call <vilib>:"NT Write Number.vi"("value"=w363, "name"=w362) -> ()  [unwired: 9 in, 1 out]
      }
      event "Test Ring": Value Change {
        # "When a test mode helper value is selected from the ring,\nset the tree item's variable to the string value"
        n250 = event-data() -> ("NewVal"=w371:u16)  [unwired: 1 in]
        n251 = property on="Test Ring" class="Ring (strict)"() -> ("Strings []"=w372:string[])  [unwired: 2 in, 2 out]
        n252 = Index Array(array=w372, index=w371) -> (element=w370:string)
        n253 = call <vilib>:"NT Write String.vi"("value"=w370, "name"=w369) -> ()  [unwired: 9 in, 1 out]
      }
      event "Rec Mode": Value Change {
        # "Update globals for recording mode and path to read log from.\nClear when logging and let NetworkTables set path for vision to\nuse."
        n254 = event-data() -> ("NewVal"=w381:enum32{"Stop", "Record", "Playback"})  [unwired: 1 in]
        n255 = global write "WPI_DashboardLogging Global.vi" "Logging Filename"(path "") -> ()
        n256 = global write "WPI_DashboardLogging Global.vi" "Recording"(w381) -> ()
        n257 = case shown="\"Playback\"" w381 {
          tunnel: w380 -> [_ w383 w391]
          tunnel: [_ _ w390] -> w378
          tunnel: [_ _ w389] -> _
          tunnel: w376 -> [_ _ w387]
          tunnel: cluster{i32, i32} {-250, 170} -> [_ _ w386]
          tunnel: [_ _ T25 {"Image Size"=TRUE, "Image Type"=TRUE, "Pixel Value"=TRUE, "ROI Information"=TRUE, "Zoom Factor"=FALSE} ("Image Information Shown:All Elements")] -> w373
          tunnel: [_ _ TRUE ("Zoom Factor")] -> w374
          frame Default {
          }
          frame "Stop", "Record" {
            # "Place Window too"
            n258 = invoke class="VI" method="FP.Close"(reference=w383) -> (reference out=w382:refnum<vi>)  [unwired: 2 in, 2 out]
            n259 = invoke class="VI" method="Abort VI"(reference=w382) -> ()  [unwired: 2 in, 3 out]
          }
          frame "Playback" {
            n260 = call "Open Playback Panel.vi"("Offset"=w386, "DB VI Ref"=w387, "Playback in"=w391) -> ("Playback out"=w388:refnum<vi>)  [unwired: 8 in]
            n261 = register-events(w388) -> (reference out=w390:refnum<event-registration>, error out=w389:errorcluster)  [unwired: 2 in]
          }
        }
        n262 = property on="Camera Image Right" class="ImageControl"("Image Information Shown"=w373, "Image Information Visible"=w374) -> ()  [unwired: 2 in, 2 out]
        n263 = property on="Camera Image" class="ImageControl"("Image Information Shown"=w373, "Image Information Visible"=w374) -> ()  [unwired: 2 in, 2 out]
        n264 = call <vilib>:"WPI_DashboardNT Log FieldName Cache.vi"("Operation"=enum16{"Lookup/Add", "Index", "Clear"}."Clear") -> ()  [unwired: 8 in, 3 out]
      }
      event Panel Close {
        w392 = enum32{"Stop", "Record", "Playback"}."Stop" ("Rec Mode")
        # "Playback window has been closed, abort"
        n265 = event-data() -> ()  [unwired: 1 in, 4 out]
        n266 = local write "Rec Mode"(w392) -> ()
        n267 = global write "WPI_DashboardLogging Global.vi" "Recording"(w392) -> ()
      }
      event Panel Close {
        # "Abort playback window and ourself"
        n268 = event-data() -> ()  [unwired: 1 in, 4 out]
        n269 = invoke class="VI" method="FP.Close"(reference=w395) -> (reference out=w394:refnum<vi>)  [unwired: 2 in, 2 out]
        n270 = invoke class="VI" method="Abort VI"(reference=w394) -> (error out=w393:errorcluster)  [unwired: 2 in, 2 out]
        n271 = invoke class="VI" method="Abort VI"(error in=w393) -> ()  [unwired: 2 in, 3 out]
      }
      event "Tree": Double Click {
        n272 = event-data() -> ("PlatMods"=w401:T27, "Tag"=w398:string)  [unwired: 1 in]
        n273 = Unbundle(w401) -> ("Shift"=w400:bool)  [unwired: 4 out]
        n274 = String Subset(string=w398, length (rest)=1 ("length (rest)")) -> (substring=w397:string)  [unwired: 1 in]
        n275 = Not(x=w400) -> (.not. x?=w399:bool)
        n276 = case shown="\"/\"" w397 {
          tunnel: w398 -> [_ w403]
          tunnel: w399 -> [_ w402]
          frame Default {
          }
          frame "/" {
            n277 = call <vilib>:"NT Update Persistence.vi"("Persistence"=w402, "Name"=w403) -> ()  [unwired: 9 in, 1 out]
          }
        }
      }
    }
  }
  n278 = while {
    tunnel: w55 -> [w405]
    i -> [w408]
    stop <- FALSE stop-if-true
    n279 = Wait (ms)(milliseconds to wait=u32 100) -> ()  [unwired: 1 out]
    n280 = case shown="\"Playback\"" "Rec Mode" {
      tunnel: w408 -> [_ _ w423]
      tunnel: [u32 2829099 ("Base Color") u32 11141120 ("Target Color") w412] -> w404
      frame "Stop", Default {
        # "Reset the color, extra updates don't cost much"
      }
      frame "Record" {
      }
      frame "Playback" {
        # "Playback"
        n281 = Quotient & Remainder(x=w423, y=u32 50 ("milliseconds to wait")) -> (x-y*floor(x/y)=w419:u32)  [unwired: 1 out]
        n282 = Divide(x=w419, y=u32 50 ("milliseconds to wait")) -> (x/y=w416:dbl)
        n283 = Multiply(x=6.283185307179586, y=w416) -> (x*y=w421:dbl)
        n284 = Sine(x=w421) -> (sin(x)=w420:dbl)
        n285 = Absolute Value(x=w420) -> (abs(x)=w413:dbl)
        n286 = call "Interpolate RGB Color.vi"("Proportion"=w413, "Target Color"=u32 30976, "Base Color"=u32 2829099) -> ("Result Color"=w412:u32)  [unwired: 8 in]
      }
    }
    n287 = property class="Pane"(reference=w405, "PaneColor"=w404) -> ()  [unwired: 1 in, 2 out]
  }
  n288 = local write "Dashboard Tab"(T2."Custom" ("Dashboard Tab")) -> ()
  n289 = property on="On/Off" class="Bool (strict)"("Visible"=w27) -> ()  [unwired: 2 in, 2 out]
  n290 = property on="Motor" class="Clust (strict)"("Visible"=w27) -> ()  [unwired: 2 in, 2 out]
  n291 = property on="Progress" class="Clust (strict)"("Visible"=w27) -> ()  [unwired: 2 in, 2 out]
  n292 = property on="Test Ring" class="Ring (strict)"("Visible"=w27) -> ()  [unwired: 2 in, 2 out]
  n293 = property on="Rev/Fwd" class="Clust (strict)"("Visible"=w27) -> ()  [unwired: 2 in, 2 out]
  n294 = while {
    tunnel: u16 1741 ("timeout ms (25000)") -> [w425]
    stop <- FALSE stop-if-true
    n295 = TCP Create Listener(10:w425) -> (0:w424:errorcluster, 3:w426:refnum<k5>)  [unwired: 4 in, 1 out]
    n296 = case shown="No Error" w424 {
      selector: w424 -> [w428 _]
      tunnel: w426 -> [w429 _]
      frame No Error {
        n297 = while {
          tunnel: w429 -> [w432]
          tunnel: w428 -> [w431]
          stop <- FALSE stop-if-true
          n298 = TCP Wait On Listener(8:w431, 11:w432) -> (0:w433:errorcluster, 4:w434:refnum<k5>)  [unwired: 2 in, 3 out]
          n299 = local write "TCP"(w434) -> ()
          n300 = case shown="Error" w433 {
            frame No Error {
            }
            frame Error {
              n301 = Wait (ms)(milliseconds to wait=u32 1000) -> ()  [unwired: 1 out]
            }
          }
        }
      }
      frame Error {
        n302 = Wait (ms)(milliseconds to wait=u32 1000) -> ()  [unwired: 1 out]
      }
    }
  }
  n303 = global write "WPI_DashboardLogging Global.vi" "Recording"(w50) -> ()
  n304 = local write "Rec Mode"(w50) -> ()
  n305 = call <vilib>:"NT Write String.vi"("value"="Select Auto", "name"="Auto Selector" ("Name")) -> ()  [unwired: 9 in, 1 out]
